vi "Get variable parm info.vi"(8 "error in (no error)":errorcluster, 9 "Token list":string[](array[string]), 10 "Query":string, 11 "Search name":string) -> (0 "error out":errorcluster, 2 "Stop button hit":bool, 3 "Fixed up query":string)   [LabVIEW 2013]
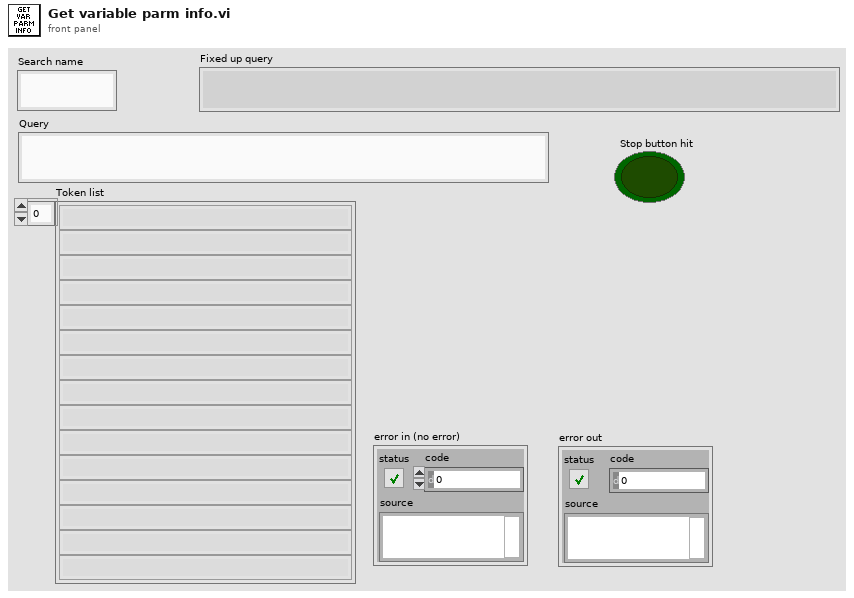
[diagram p1: front panel]
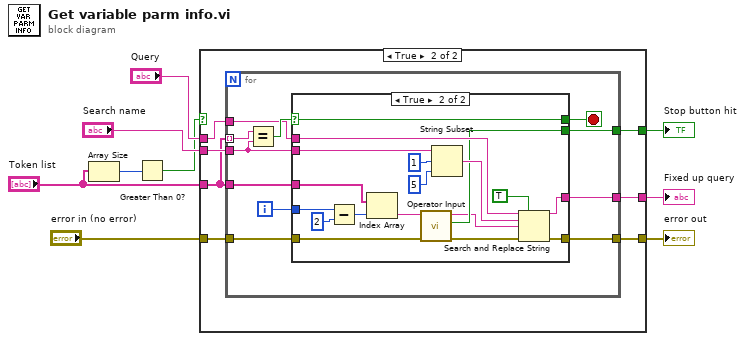
[diagram p0: block diagram]
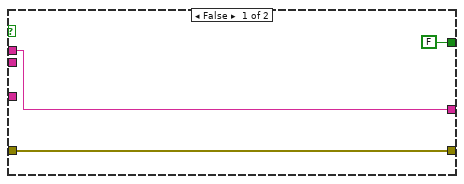
[diagram p2: hidden frame]
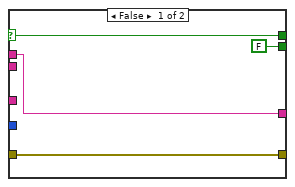
[diagram p3: hidden frame]
diagram:
  n1 = Array Size(array="Token list") -> (size(s)=w3:i32)
  n2 = Greater Than 0?(x=w3) -> (x > 0?=w2:bool)
  n3 = case shown="True" w2 {
    tunnel: "Search name" -> [_ w19]
    tunnel: [w12 w18] -> w8
    tunnel: "error in (no error)" -> [w12 w17]
    tunnel: "Query" -> [w11 w16]
    tunnel: [w11 w15] -> w5
    tunnel: "Token list" -> [_ w14]
    tunnel: [FALSE ("Stop button hit") w13] -> w1
    frame False {
    }
    frame True {
      n4 = for {
        tunnel: w14 -> [w30] mode=indexing
        tunnel: w14 -> [w28]
        tunnel: w16 -> [w26]
        tunnel: [w24] -> w15
        tunnel: w17 -> [w23]
        tunnel: [w22] -> w18
        tunnel: w19 -> [w21]
        tunnel: [w20] -> w13
        i -> [w27]
        stop <- w25 stop-if-true
        n5 = Equal?(x=w30, y=w21) -> (x = y?=w29:bool)
        n6 = case shown="True" w29 {
          selector: w29 -> [w33 w43]
          tunnel: w28 -> [_ w52]
          tunnel: w27 -> [_ w51]
          tunnel: w26 -> [w34 w47]
          tunnel: [w34 w44] -> w24
          tunnel: [w33 w43] -> w25
          tunnel: w23 -> [w32 w42]
          tunnel: [w32 w41] -> w22
          tunnel: w21 -> [_ w40]
          tunnel: [FALSE ("Stop button hit") w36] -> w20
          frame False {
          }
          frame True {
            n7 = Subtract(x=w51, y=2) -> (x-y=w49:i32)
            n8 = Index Array(array=w52, index=w49) -> (element=w48:string)
            n9 = call "Operator Input.vi"("error in (no error)"=w42, "Message"=w48) -> ("error out"=w46:errorcluster, "Stop button hit"=w36:bool, "Response"=w35:string)  [unwired: 7 in]
            n10 = String Subset(string=w40, offset (0)=1, length (rest)=5 ("length (rest)")) -> (substring=w37:string)
            n11 = Search and Replace String(replace all?=TRUE ("replace all? (F)"), input string=w47, search string=w37, replace string=w35, error in=w46) -> (result string=w44:string, error out=w41:errorcluster)  [unwired: 3 in, 2 out]
          }
        }
      }
    }
  }
  "error out" <- w8
  "Fixed up query" <- w5
  "Stop button hit" <- w1
